vi "SLM_display.vi"(10 "weight SLMB":dbl=1.0, 11 "weight SLM A":dbl=1.0) -> ()   [LabVIEW 2015]
uses:
  <userlib>/TAM_Program/TAM Sub VIs.llb/BaseHologramGlobal.vi
panel:
  in  "?":bool
  in  "no of columns & rows":i32=600
  in  "modes":T1(array[cluster])=[{"type"=enum."LG mode", "m or L"=-2, "n or p"=0, "weight"=0.7071, "phase"=0.0}, {"type"=enum."LG mode", "m or L"=2, "n or p"=0, "weight"=0.7071, "phase"=0.0}]
  in  "Enc or LG":bool
  in  "Encoding":cluster{"d":dbl, "y0":dbl, "y1":dbl}
  out "?":dbl[][](graph)
  out "max value":dbl=0.0002545111260339989
  in  "Load global\nbase parameters?":bool=TRUE
  in  "Base hologram parameters":T2={"x centre A (m)"=0.00023877834010536838, "y centre A (m)"=-1.0895093102686923e-05, "x angle A (mrad)"=10.0, "y angle A (mrad)"=0.0, "f lens A (m)"=1000000.0, "x centre B (m)"=-0.00031192399117047087, "y centre B (m)"=-0.00028507383868835634, "x angle B (mrad)"=10.0, "y angle B (mrad)"=0.0, "f lens B (m)"=1000000.0} {"f lens B (m)" format="%_3g"; "y angle B (mrad)" format="%_8g"; "x angle B (mrad)" format="%_8g"; "y centre B (m)" format="%_8p"; "x centre B (m)" format="%_8p"; "f lens A (m)" format="%_3g"; "y angle A (mrad)" format="%_8g"; "x angle A (mrad)" format="%_8g"; "y centre A (m)" format="%_8p"; "x centre A (m)" format="%_8p"}
  in  "beam waist w0 (m)":dbl=0.0005 format="%_3p"
  out "Hologram A":u8[][](graph)
  # "Set global\nbase parameters?"
  # "to account for \nunequal efficiencies,\nset to 1 if not intensity masking"
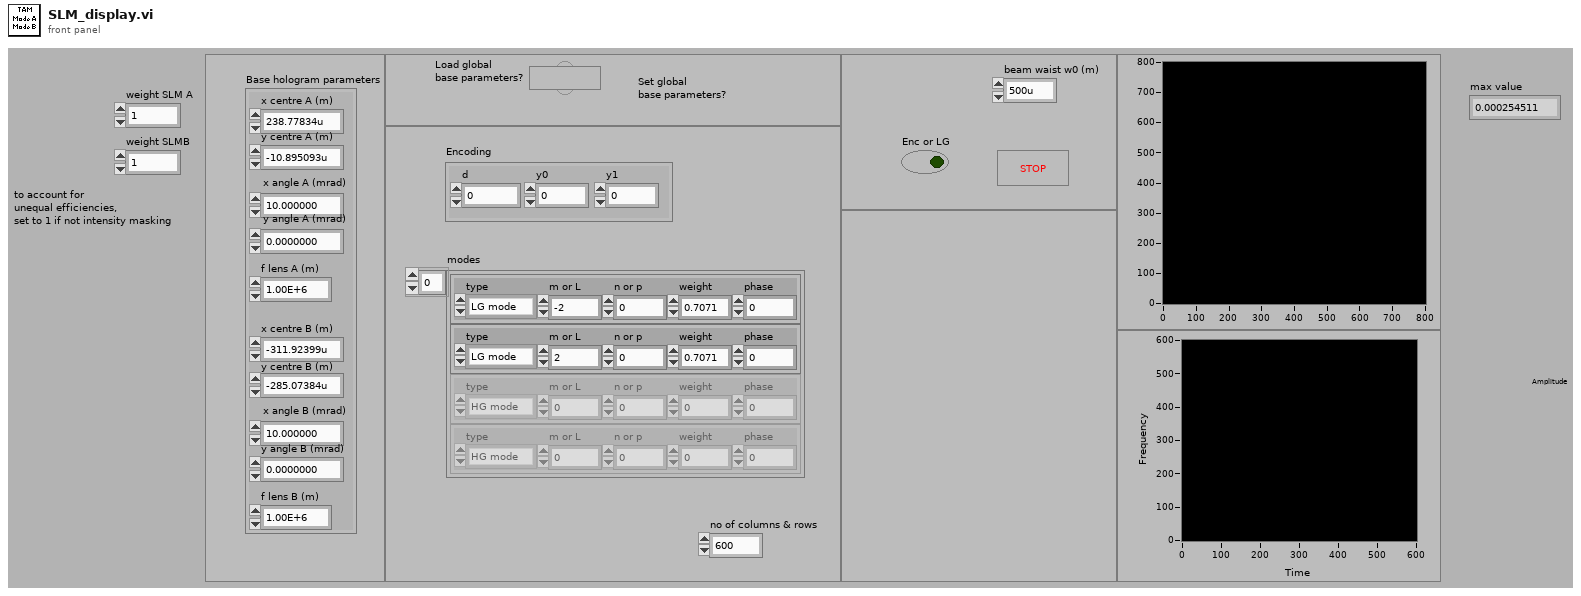
[diagram p1: front panel]
types:
  T1 = cluster{"type":enum16{"HG mode", "LG mode"}, "m or L":i32, "n or p":i32, "weight":dbl, "phase":dbl}[]
  T2 = cluster{"x centre A (m)":dbl, "y centre A (m)":dbl, "x angle A (mrad)":dbl, "y angle A (mrad)":dbl, "f lens A (m)":dbl, "x centre B (m)":dbl, "y centre B (m)":dbl, "x angle B (mrad)":dbl, "y angle B (mrad)":dbl, "f lens B (m)":dbl}
  T3 = cluster{"amplitude matrix":cdb[][], "number of columns in amplitude matrix":i32, "number of rows in amplitude matrix":i32, "represented width (in m)":dbl, "represented height (in m)":dbl, "wavelength (in m)":dbl}
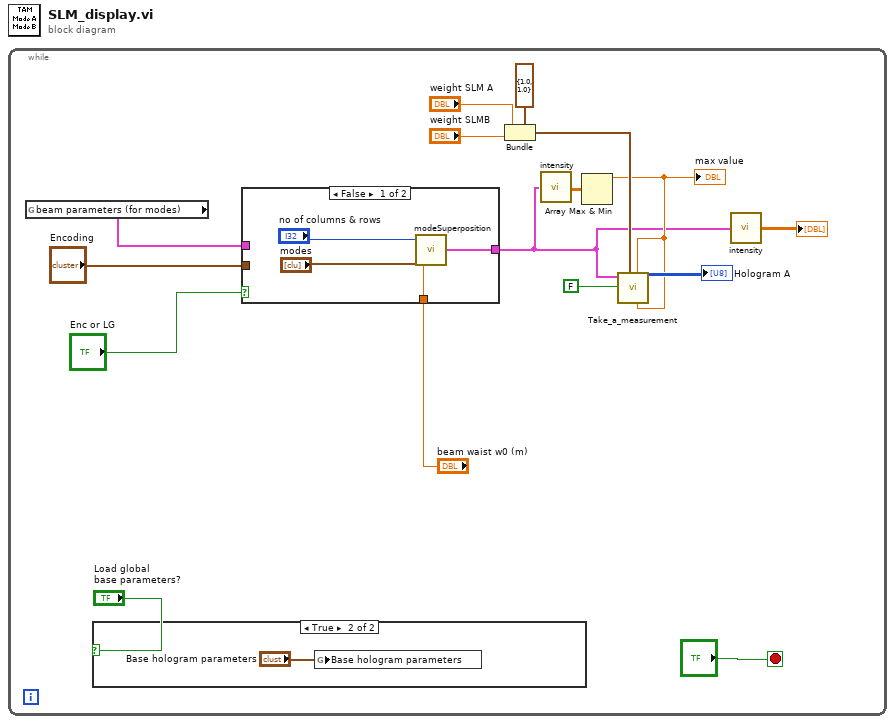
[diagram p0: block diagram]
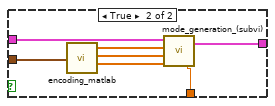
[diagram p2: hidden frame]
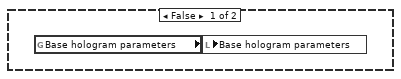
[diagram p3: hidden frame]
diagram:
  n1 = while {
    stop <- "?" stop-if-true
    n2 = global read "BaseHologramGlobal.vi" "beam parameters (for modes)"() -> (w4:T3)
    n3 = case shown="True" "Load global\nbase parameters?" {
      frame False {
        n4 = global read "BaseHologramGlobal.vi" "Base hologram parameters"() -> (w28:T2)
        n5 = local write "Base hologram parameters"(w28) -> ()
      }
      frame True {
        n6 = global write "BaseHologramGlobal.vi" "Base hologram parameters"("Base hologram parameters") -> ()
      }
    }
    n7 = case shown="False" "Enc or LG" {
      tunnel: "beam waist w0 (m)" -> [w17 w27]
      tunnel: [w20 w26] -> w6
      tunnel: w4 -> [_ w25]
      tunnel: "Encoding" -> [_ w21]
      frame False {
        n8 = call <userlib>:"modeSuperposition.vi"("modes"="modes", "no of columns & rows"="no of columns & rows", "beam waist w0 (in m; default 1E-4 = 0.1mm)"=w17) -> ("mode superposition"=w20:T3)  [unwired: 4 in]
      }
      frame True {
        n9 = call "encoding_matlab.vi"("Encoding"=w21) -> ("modes"=w24:dbl[], "coeffs"=w23:dbl[], "phase"=w22:dbl[])
        n10 = call "mode_generation_(subvi).vi"("beam waist w0 (m) in"=w27, "phase"=w22, "coeffs"=w23, "modes"=w24, "beam parameters in"=w25) -> ("mode encoding"=w26:T3)
      }
    }
    n11 = Bundle(cluster=cluster{"weight A":dbl, "weight B":dbl} {"weight A"=1.0, "weight B"=1.0} ("Weights for SLM"), "weight A"="weight SLM A", "weight B"="weight SLMB") -> (w14:cluster{"weight A":dbl, "weight B":dbl})
    n12 = call <userlib>:"intensity.vi"("beam cluster"=w6) -> ("intensity matrix"=w12:dbl[][])
    n13 = Array Max & Min(array=w12) -> (max value=w10:dbl)  [unwired: 3 out]
    "max value" <- w10
    n14 = call <userlib>:"Take_a_measurement.vi"("ref intensity B"=w10, "ref intensity A"=w10, "Use ref. intensity"=FALSE, "Weights for SLM"=w14, "Mode A"=w6) -> ("Hologram A"=→"Hologram A":u8[][])  [unwired: 5 in, 1 out]
    n15 = call <userlib>:"intensity.vi"("beam cluster"=w6) -> ("intensity matrix"=→"?":dbl[][])
  }
